vi "整形转浮点CDAB.vi"(11 "数组":u16[](array[numeric]) format="%04xH") -> (3 "CDAB":sgl[](array[numeric]))   [LabVIEW 2016, in "斯坦道功率测流.lvlib"]
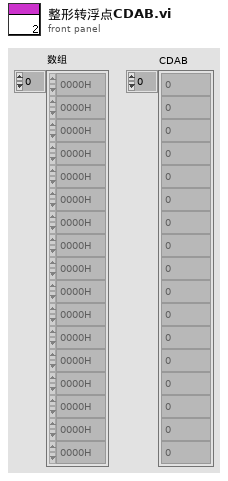
[diagram p1: front panel]
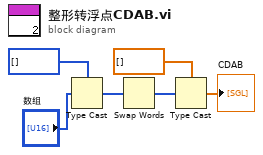
[diagram p0: block diagram]
diagram:
  n1 = Type Cast(type=u32[] [], x="数组") -> (*(type *) &x=w2:u32[])
  n2 = Swap Words(1:w2) -> (0:w1:u32[])
  n3 = Type Cast(type=sgl[] [], x=w1) -> (*(type *) &x=→"CDAB":sgl[])
